vi "Send ppanel_stream_TTTR.vi"(2 "Correlation_settings":T1 {"Lag Settings"."time_start" items=["1 ps"=1, "10 ps"=10, "100 ps"=100, "1 ns"=1000, "10 ns"=10000, "100 ns"=100000, "1 us"=1000000, "10 us"=10000000, "100 us"=100000000, "1 ms"=1000000000, "10 ms"=10000000000, "100 ms"=100000000000, "1 s"=1000000000000, "10 s"=10000000000000, "100 s"=100000000000000]; "Lag Settings"."time_end" items=["1 ps"=1, "10 ps"=10, "100 ps"=100, "1 ns"=1000, "10 ns"=10000, "100 ns"=100000, "1 us"=1000000, "10 us"=10000000, "100 us"=100000000, "1 ms"=1000000000, "10 ms"=10000000000, "100 ms"=100000000000, "1 s"=1000000000000, "10 s"=10000000000000, "100 s"=100000000000000]}, 4 "Record Type":T4, 5 "stop_fifo_event":refnum<event-registration>, 6 "acq_time":i32, 7 "Message Priority (Normal)":T6=enum."Normal", 8 "error in (no error)":errorcluster, 9 "action_for_records":T5, 10 "fifo_stream_path":path, 11 "Message Enqueuer":refnum<class "Message Enqueuer.lvclass">) -> (0 "error out":errorcluster, 3 "Message Enqueuer out":refnum<class "Message Enqueuer.lvclass">)   [LabVIEW 2015, in "ppanel_stream_TTTR Msg.lvclass"]
doc: "This VI sends the message to an actor."
uses:
  ppanel_stream_TTTR Msg.lvclass
  <vilib>/ActorFramework/Message Enqueuer/Message Enqueuer.lvclass
  <vilib>/ActorFramework/Message Enqueuer/Message Priority.ctl
  Hydraharp/hydraharp/hydraharp_action_on_records.ctl
  record_type.ctl
  Hydraharp/hydraharp_panel/hpanel_correlation_settings.ctl
  Hydraharp/hydraharp/hydraharp_correlation_lag_settings.ctl
  Hydraharp/hydraharp/hydraharp_time_decades.ctl
  ppanel_stream_TTTR Msg.lvclass/ppanel_stream_TTTR Msg.ctl
  <vilib>/ActorFramework/Message Enqueuer/Message Enqueuer.lvclass/Message Enqueuer.ctl
  <vilib>/ActorFramework/Message Priority Queue/Priority Enqueue.vi
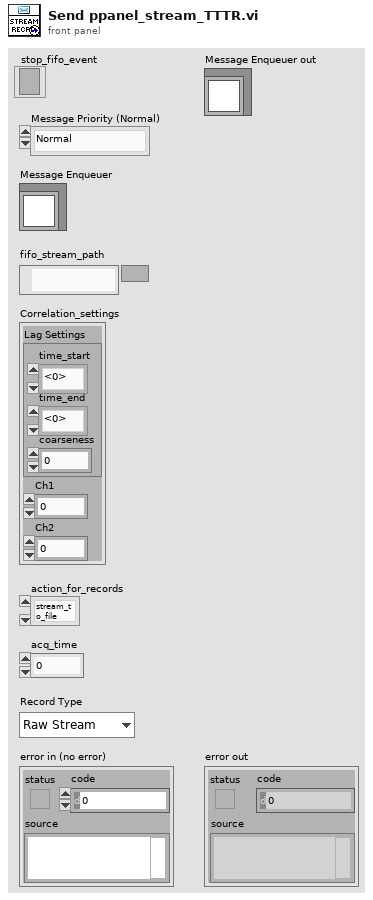
[diagram p1: front panel]
types:
  T1 = typedef "hpanel_correlation_settings.ctl" = cluster{"Lag Settings":T2, "Ch1":u8, "Ch2":u8}
  T2 = typedef "hydraharp_correlation_lag_settings.ctl" = cluster{"time_start":T3, "time_end":T3, "coarseness":i64}
  T3 = typedef "hydraharp_time_decades.ctl" = i64
  T4 = typedef "record_type.ctl" = enum16{"Raw Stream", "Processed Records (hdf5)"}
  T5 = typedef "hydraharp_action_on_records.ctl" = enum16{"stream_to_file", "correlate", "stream to file and correlate"}
  T6 = typedef "Actor Framework.lvlib/Message Enqueuer.lvclass/Message Priority.ctl" = enum16{"Low", "Normal", "High"}
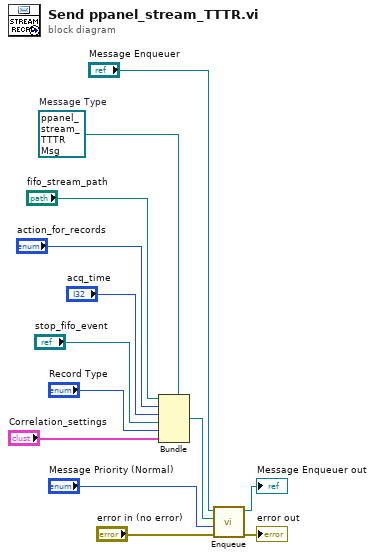
[diagram p0: block diagram]
diagram:
  w10 = refnum<class "ppanel_stream_TTTR Msg.lvclass"> refnum  # Message Type
  n1 = Bundle(cluster=w10, "fifo_stream_path", "action_for_records", "acq_time", "stop_fifo_event", "Record Type", "Correlation_settings") -> (w9:refnum<class "ppanel_stream_TTTR Msg.lvclass">)
  n2 = call <vilib>:"Enqueue.vi"("error in (no error)"="error in (no error)", "Message Priority (Normal)"="Message Priority (Normal)", "Message"=w9, "Message Enqueuer in"="Message Enqueuer") -> ("error out"=→"error out":errorcluster, "Message Enqueuer out"=→"Message Enqueuer out":refnum<class "Message Enqueuer.lvclass">)  [unwired: 6 in]
